vi "Add or replace Obj.vi"(8 "error in (no error)":errorcluster, 10 "Analyze Obj":refnum<class "Analyze BaseClass.lvclass">, 11 "Analyze Compound Analysis Base in":refnum<class "Analyze Compound Analysis Base.lvclass">) -> (0 "error out":errorcluster, 3 "Analyze Compound Analysis Base out":refnum<class "Analyze Compound Analysis Base.lvclass">)   [LabVIEW 2014, in "Analyze.lvlib" / "Analyze Compound Analysis Base.lvclass"]
uses:
  Analyze Compound Analysis Base.lvclass
  Analyze BaseClass/Analyze BaseClass/Analyze BaseClass.lvclass
  Analyze Compound Analysis Base.lvclass/Analyze Compound Analysis Base.ctl
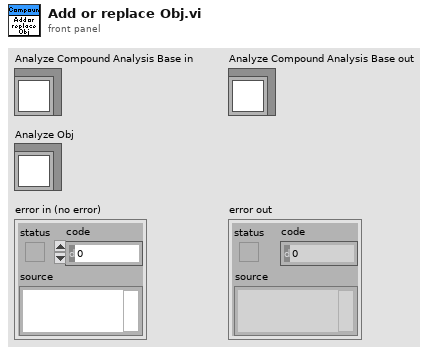
[diagram p1: front panel]
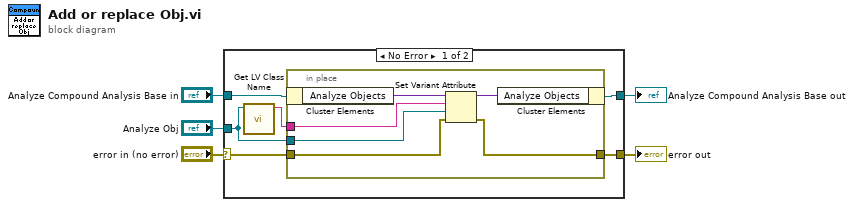
[diagram p0: block diagram]
diagram:
  n1 = case shown="No Error" "error in (no error)" {
    selector: "error in (no error)" -> [w8 w19]
    tunnel: [w7 w19] -> w3
    tunnel: [w6 w18] -> w4
    tunnel: "Analyze Compound Analysis Base in" -> [w11 w18]
    tunnel: "Analyze Obj" -> [w9 _]
    frame No Error {
      n2 = call <vilib>:"Get LV Class Name.vi"("object"=w9) -> ("class name"=w10:string)  [unwired: 9 in, 1 out]
      n3 = in-place {
        in-place-border: w10 -> [w17]
        in-place-border: w9 -> [w16]
        in-place-border: w8 -> [w13]
        in-place-border: [w12] -> w7
        n4 = in-place-cluster #1(w11) -> ("Analyze Objects"=w15:variant)
        n5 = Set Variant Attribute(Variant=w15, name=w17, value=w16, error in=w13) -> (Variant out=w14:variant, error out=w12:errorcluster)  [unwired: 1 out]
        n6 = in-place-cluster #1("Analyze Objects"=w14) -> (w6:refnum<class "Analyze Compound Analysis Base.lvclass">)
      }
    }
    frame Error {
    }
  }
  "error out" <- w3
  "Analyze Compound Analysis Base out" <- w4
